vi "Write PRODUCTOS.vi"(8 "error in (no error)":errorcluster, 10 "PRODUCTOS":refnum<vi>, 11 "UI_CAFÉ_MEX_ESP in":refnum<class "UI_CAFÉ_MEX_ESP.lvclass">) -> (0 "error out":errorcluster, 3 "UI_CAFÉ_MEX_ESP out":refnum<class "UI_CAFÉ_MEX_ESP.lvclass">)   [LabVIEW 2019, in "DATA_UI_CAFÉ_MEX_ESP.lvlib" / "UI_CAFÉ_MEX_ESP.lvclass"]
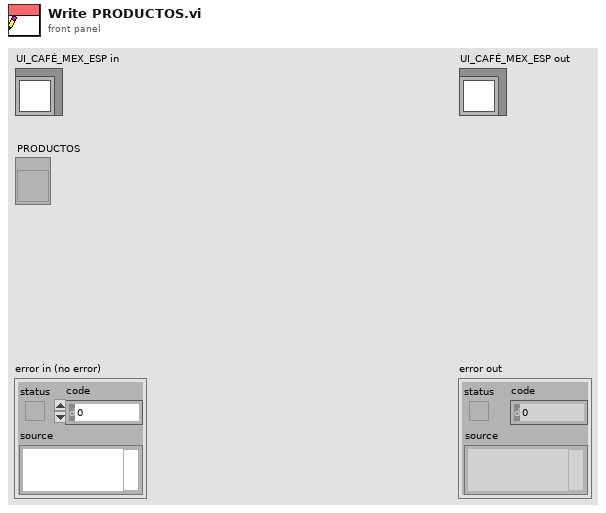
[diagram p1: front panel]
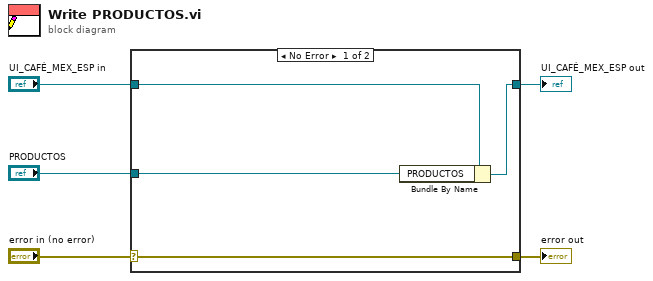
[diagram p0: block diagram]
diagram:
  n1 = case shown="No Error" "error in (no error)" {
    selector: "error in (no error)" -> [w9 w10]
    tunnel: [w9 w10] -> w4
    tunnel: [w7 w11] -> w2
    tunnel: "UI_CAFÉ_MEX_ESP in" -> [w8 w11]
    tunnel: "PRODUCTOS" -> [w6 _]
    frame No Error {
      n2 = Bundle By Name(cluster=w8, "PRODUCTOS"=w6) -> (w7:refnum<class "UI_CAFÉ_MEX_ESP.lvclass">)
    }
    frame Error {
    }
  }
  "error out" <- w4
  "UI_CAFÉ_MEX_ESP out" <- w2
